vi "Open SMO.vi"(8 "error in (no error)":errorcluster, 11 "Instrument in":refnum<class "Instrument.lvclass">) -> (0 "error out":errorcluster, 3 "Instrument out":refnum<class "Instrument.lvclass">)   [LabVIEW 2019, in "Instrument.lvclass"]
uses:
  Instrument.lvclass
  Instrument.lvclass/Instrument.ctl
  <userlib>/LevyLab/RemoteControl/RemoteControl.lvclass
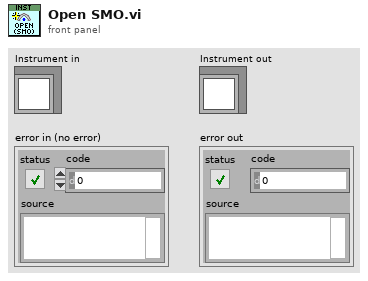
[diagram p1: front panel]
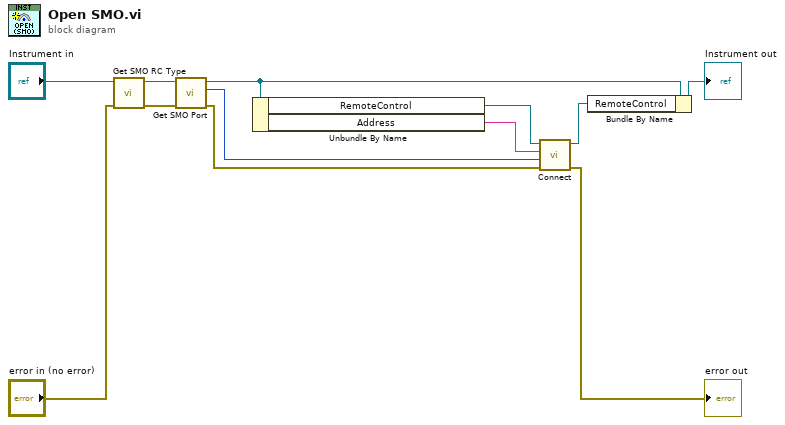
[diagram p0: block diagram]
diagram:
  n1 = call-dynamic "Get SMO RC Type.vi"("error in (no error)"="error in (no error)", "Instrument in"="Instrument in") -> ("error out"=w4:errorcluster, "Instrument out"=w3:refnum<class "Instrument.lvclass">)  [unwired: 7 in, 1 out]
  n2 = call-dynamic "Get SMO Port.vi"("error in (no error)"=w4, "Instrument in"=w3) -> ("error out"=w12:errorcluster, "Port"=w2:u16, "Instrument out"=w11:refnum<class "Instrument.lvclass">)  [unwired: 7 in]
  n3 = Unbundle By Name(w11) -> ("RemoteControl"=w7:refnum<class "RemoteControl.lvclass">, "Address"=w1:string)
  n4 = call <userlib>:"Connect.vi"("error in (no error)"=w12, "Port"=w2, "address"=w1, "RemoteControl in"=w7) -> ("error out"=→"error out":errorcluster, "RemoteControl out"=w8:refnum<class "RemoteControl.lvclass">)  [unwired: 6 in]
  n5 = Bundle By Name(cluster=w11, "RemoteControl"=w8) -> (→"Instrument out":refnum<class "Instrument.lvclass">)
